vi "Actor Core.vi"(8 "error in":errorcluster, 11 "Monitor in":refnum<class "Classic Monitor.lvclass">) -> (0 "error out":errorcluster, 3 "Actor out":refnum<class "Actor.lvclass">)   [LabVIEW 2023, in "Monitored Actor.lvlib" / "Classic Monitor.lvclass"]
doc: "(<B>Filename</B>: Actor Framework.lvlib:Actor.lvclass:Actor Core.vi)\n\nReceives messages to the actor, reacts to them, and initiates any error handling that may shut the actor down.\n\nDescendant classes may override this VI to append parallel tasks for the actor to complete while it handles messages. Overrides use the Call Parent Method node."
uses:
  Classic Monitor.lvclass
  C:/Users/Public/Documents/Development/builds/Engine/Actor Framework.lvlibp/1abvi3w/vi.lib/ActorFramework/Actor/Actor.lvclass
  builds/Engine/Actor Framework.lvlibp/1abvi3w/vi.lib/ActorFramework/Actor/Actor.lvclass
  Monitor Data/Monitor Data.lvclass
  builds/Engine/Actor Framework.lvlibp/1abvi3w/vi.lib/ActorFramework/Message Enqueuer/Message Enqueuer.lvclass
  Classic Monitor.lvclass/Classic Monitor.ctl
  builds/Engine/Actor Framework.lvlibp/1abvi3w/vi.lib/ActorFramework/Time-Delayed Send Message/Time-Delay Override Options.ctl
  Orphan Detector/Orphan Detector/Orphan Detector.lvclass
  Actor Monitor/Actor Monitor Messages/Ping Actor Msg/Ping Actor Msg.lvclass
  C:/Users/Public/Documents/Development/builds/Engine/Actor Framework.lvlibp/1abvi3w/vi.lib/ActorFramework/Message/Message.lvclass
  Actor Monitor/Actor Monitor/Actor Monitor.lvclass
  Actor Monitor/Actor Monitor Messages/Manually Remove Actor Msg/Manually Remove Actor Msg.lvclass
  Monitor Messages/Log Messages Msg/Log Messages Msg.lvclass
  builds/Engine/Actor Framework.lvlibp/1abvi3w/vi.lib/ActorFramework/Stop Msg/Stop Msg.lvclass
  builds/Engine/Actor Framework.lvlibp
panel:
  in  "Monitored Actors":string[](tree)
  in  "Stop Actor":bool
  in  "Show Actor Core":bool
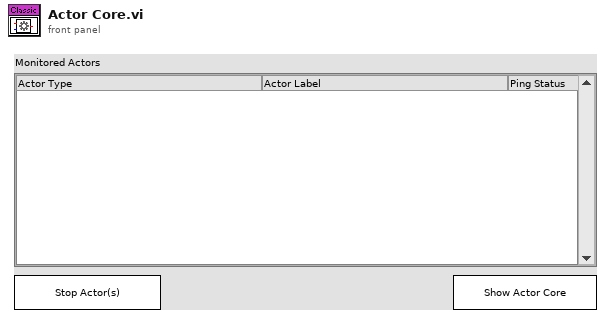
[diagram p1: front panel]
types:
  T1 = cluster{"Monitor Data":refnum<class "Monitor Data.lvclass">, "Changed Actor Q":refnum<class "Message Enqueuer.lvclass">}
  T2 = enum32{"Invalid", "Standard", "Closed", "Hidden", "Minimized", "Maximized"}
  T3 = cluster{"left":i16, "top":i16, "right":i16, "bottom":i16}
  T4 = typedef "Actor Framework.lvlibp/Time-Delay Override Options.ctl" = enum16{"Send next copy now", "Skip next scheduled copy", "Send next copy now and stop all further copies", "Stop all further copies"}
  T5 = enum8{"Enabled", "Disabled", "Disabled and Grayed Out"}
  T6 = typedef "LVRectTypeDef.ctl" = cluster{"Left":i16, "Top":i16, "Right":i16, "Bottom":i16}
  T7 = typedef "LVPoint32TypeDef.ctl" = cluster{"Horizontal":i32, "Vertical":i32}
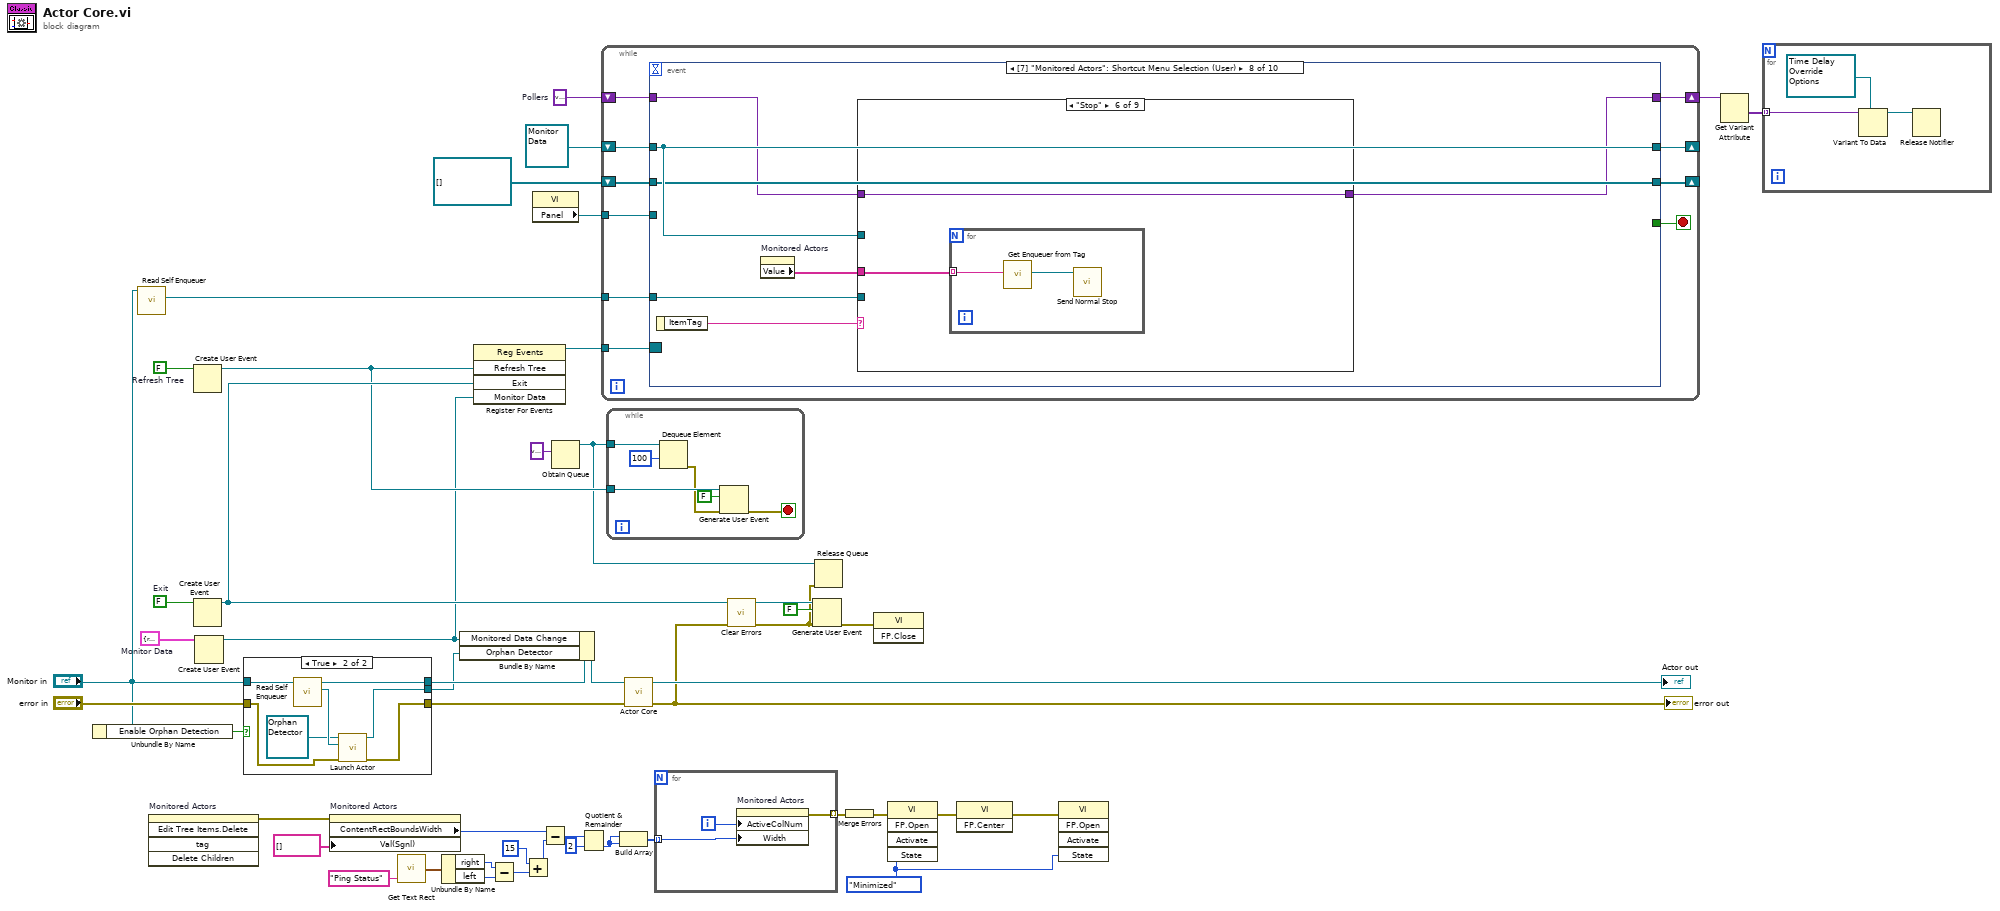
[diagram p0: block diagram]
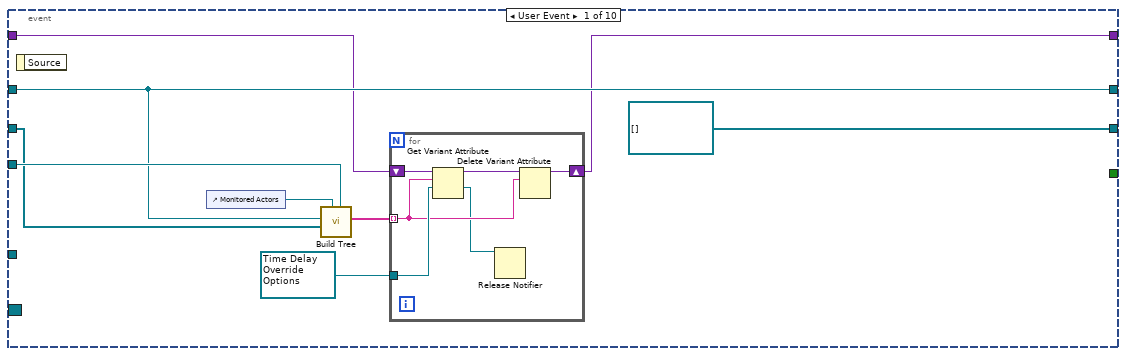
[diagram p3: hidden frame]
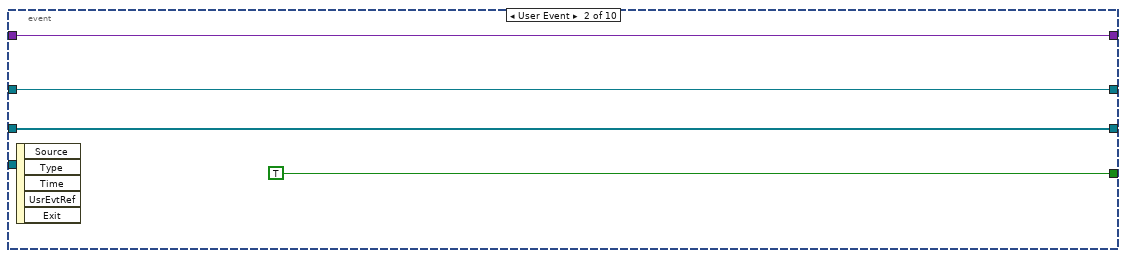
[diagram p4: hidden frame]
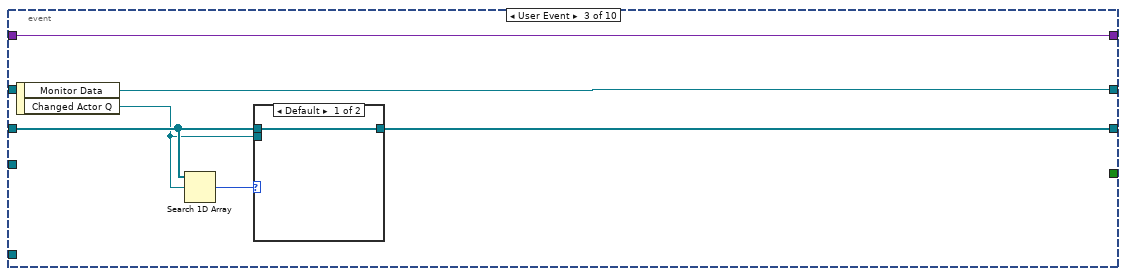
[diagram p5: hidden frame]
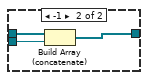
[diagram p6: hidden frame]
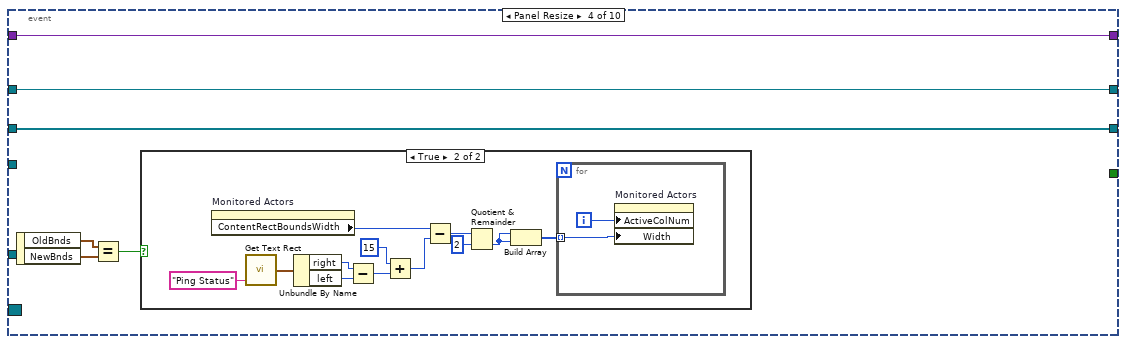
[diagram p7: hidden frame]
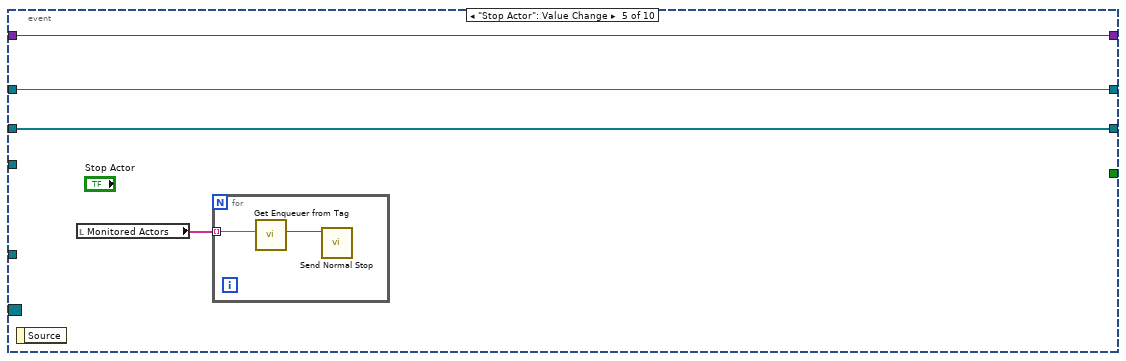
[diagram p9: hidden frame]
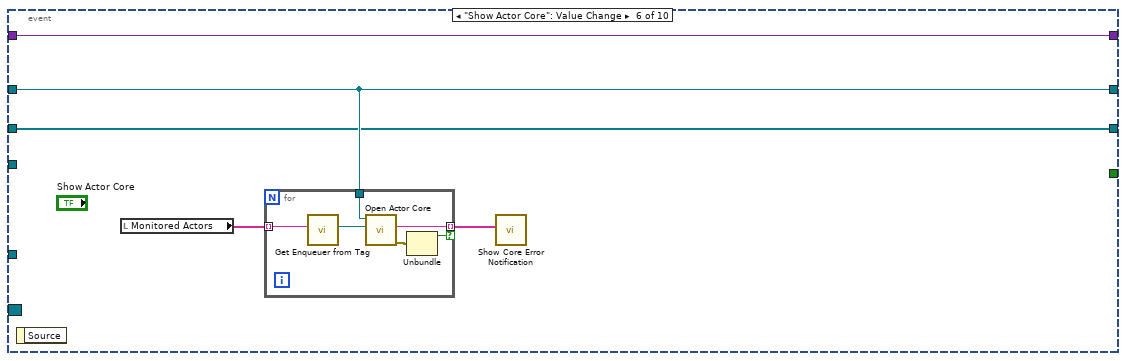
[diagram p10: hidden frame]
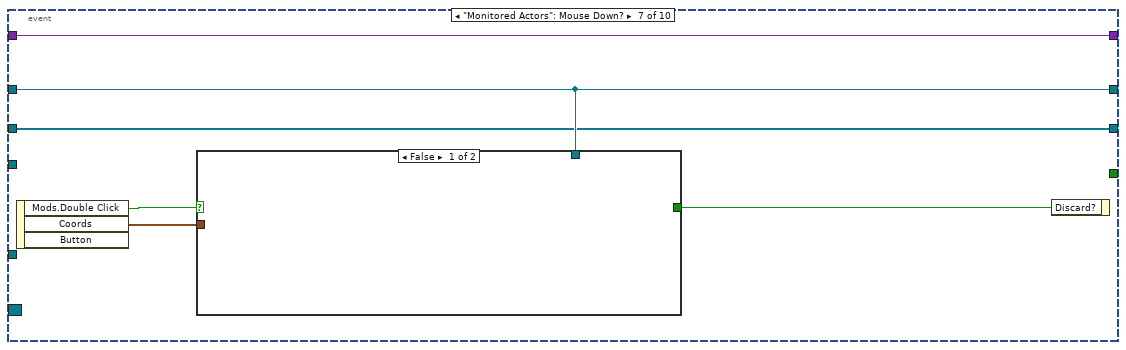
[diagram p11: hidden frame]
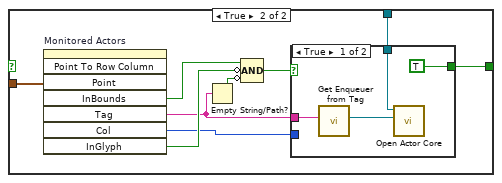
[diagram p12: hidden frame]
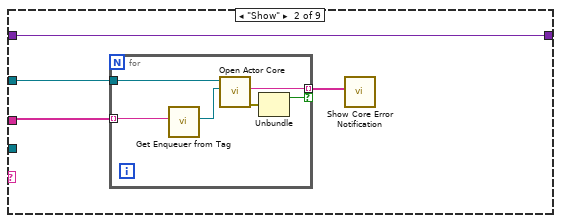
[diagram p15: hidden frame]
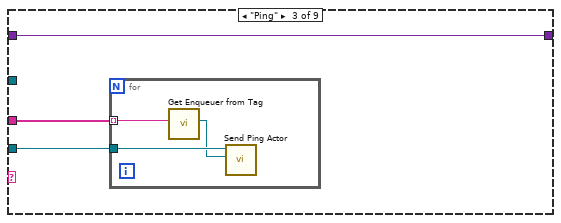
[diagram p16: hidden frame]
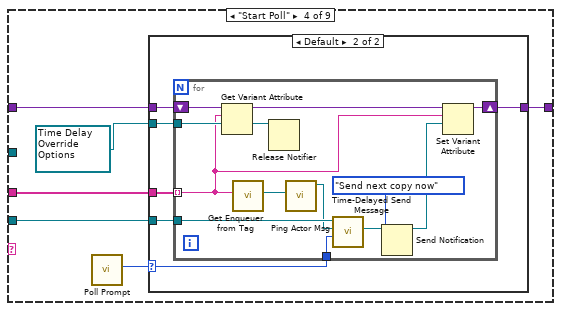
[diagram p17: hidden frame]
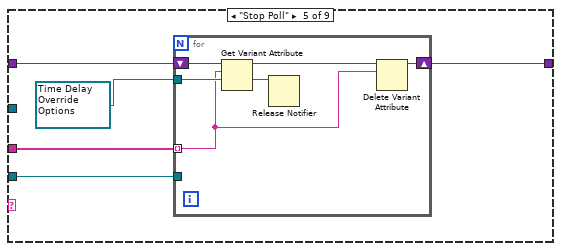
[diagram p19: hidden frame]
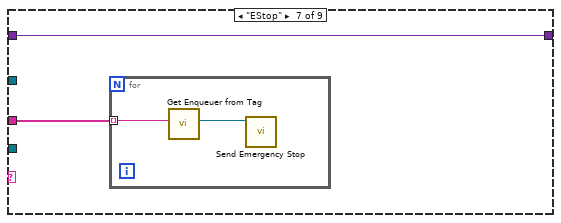
[diagram p20: hidden frame]
diagram:
  w4 = variant  # Pollers
  w15 = T1 {"Monitor Data"=refnum, "Changed Actor Q"=refnum}  # Monitor Data
  w20 = FALSE  # Refresh Tree
  w1 = T2."Minimized" ("State")
  w32 = FALSE  # Exit
  n1 = Unbundle By Name("Monitor in") -> ("Enable Orphan Detection"=w5:bool)
  n2 = call "Read Self Enqueuer.vi"("Actor"="Monitor in") -> ("Self Enqueuer"=w26:refnum<class "Message Enqueuer.lvclass">)  [unwired: 10 in]
  n3 = invoke on="Monitored Actors" class="Tree (strict)" method="Edit Tree Items.Delete"() -> (error out=w11:errorcluster)  [unwired: 5 in, 4 out]
  n4 = Create User Event(user event datatype=w20) -> (user event=w19:refnum<user-event>)  [unwired: 1 in, 1 out]
  n5 = Create User Event(user event datatype=w32) -> (user event=w31:refnum<user-event>)  [unwired: 1 in, 1 out]
  n6 = Create User Event(user event datatype=w15) -> (user event=w14:refnum<user-event>)  [unwired: 1 in, 1 out]
  n7 = case shown="True" w5 {
    tunnel: "error in" -> [w48 w51]
    tunnel: [w48 w50] -> w10
    tunnel: [w49 w54] -> w9
    tunnel: "Monitor in" -> [w49 w54]
    tunnel: [_ w52] -> w8
    frame False {
    }
    frame True {
      n8 = call "Read Self Enqueuer.vi"("Actor"=w54) -> ("Self Enqueuer"=w55:refnum<class "Message Enqueuer.lvclass">)  [unwired: 10 in]
      n9 = call "Launch Actor.vi"("error in (no error)"=w51, "Actor-to-Caller Enqueuer"=w55, "Actor"=refnum<class "Orphan Detector.lvclass"> refnum ("Classic Monitor.lvlib:Orphan Detector.lvclass")) -> ("error out"=w50:errorcluster, "Caller-To-Actor Enqueuer"=w52:refnum<class "Message Enqueuer.lvclass">)  [unwired: 7 in]
    }
  }
  n10 = property on="Monitored Actors" class="Tree (strict)"(error in=w11, "Val(Sgnl)"=string[] [] ("Value (Signaling)")) -> ("ContentRectBoundsWidth"=w45:i32)  [unwired: 1 in, 2 out]
  n11 = call <vilib>:"Get Text Rect.vi"("text"="Ping Status") -> ("rect"=w43:T3)  [unwired: 8 in]
  n12 = Unbundle By Name(w43) -> ("right"=w42:i16, "left"=w41:i16)
  n13 = Bundle By Name(cluster=w9, "Monitored Data Change"=w14, "Orphan Detector"=w8) -> (w29:refnum<class "Classic Monitor.lvclass">)
  n14 = register-events(w19, w31, w14) -> (reference out=w33:refnum<event-registration>)  [unwired: 2 in, 1 out]
  n15 = Subtract(x=w42, y=w41) -> (x-y=w40:i16)
  n16 = Add(x=i16 15, y=w40) -> (x+y=w37:i16)
  n17 = property class="VI"() -> ("Panel"=w27:refnum<vi>)  [unwired: 2 in, 2 out]
  n18 = Subtract(x=w45, y=w37) -> (x-y=w39:i32)
  n19 = Obtain Queue(element data type=variant) -> (queue out=w16:refnum<queue>)  [unwired: 4 in, 2 out]
  n20 = Quotient & Remainder(x=w39, y=2) -> (floor(x/y)=w35:i32)  [unwired: 1 out]
  n21 = while {
    tunnel: w33 -> [w65]
    shift-right: [w63] -> _
    shift-left: refnum<class "Monitor Data.lvclass"> refnum ("Monitor Data") -> [w62]
    tunnel: w27 -> [w61]
    tunnel: w26 -> [w60]
    shift-right: [w59] -> _
    shift-left: refnum<class "Message Enqueuer.lvclass">[] [] -> [w58]
    shift-right: [w57] -> w3
    shift-left: w4 -> [w56]
    stop <- w64 stop-if-true
    n22 = event shown="[7] \"Monitored Actors\": Shortcut Menu Selection (User)" {
      selector: w65 -> [_ _ _ _ _ _ _ _ _ _]
      dyn-events: _ -> [_ _ _ _ _ _ _ _ _ _]
      timeout: _ -> [_ _ _ _ _ _ _ _ _ _]
      tunnel: [_ TRUE _ _ _ _ _ _ _ _] -> w64
      tunnel: [w73 w83 w90 w100 w118 w124 w137 w157 w242 w259] -> w63
      tunnel: w62 -> [w73 w83 _ w100 w118 w124 w137 w157 w242 w259]
      tunnel: w61 -> [w74 _ _ _ _ _ _ _ _ _]
      tunnel: w60 -> [_ _ _ _ _ _ _ w154 _ _]
      tunnel: [refnum<class "Message Enqueuer.lvclass">[] [] w82 w89 w96 w116 w123 w133 w153 w243 w261] -> w59
      tunnel: w58 -> [w66 w82 w88 w96 w116 w123 w133 w153 w243 w261]
      tunnel: [w67 w81 w85 w95 w115 w121 w132 w151 w236 w252] -> w57
      tunnel: w56 -> [w68 w81 w85 w95 w115 w121 w132 w152 w236 w252]
      event User Event {
        w69 = refnum<notifier> refnum items=["Send next copy now", "Skip next scheduled copy", "Send next copy now and stop all further copies", "Stop all further copies"] ("Delivery Notifier")
        n23 = event-data() -> ()  [unwired: 1 in, 1 out]
        n24 = control-ref of="Monitored Actors"() -> (w72:refnum<vi>)
        n25 = call "Build Tree.vi"("Panel"=w74, "Tree"=w72, "Changed Actors"=w66, "Monitor Data"=w73) -> ("Stopped Actors"=w70:string[])  [unwired: 7 in]
        n26 = for {
          tunnel: w70 -> [w77] mode=indexing
          shift-right: [w76] -> w67
          shift-left: w68 -> [w80]
          tunnel: w69 -> [w79]
          n27 = Get Variant Attribute(Variant=w80, name=w77, default value (empty Variant)=w79) -> (duplicate Variant=w78:variant, value=w75:refnum<notifier>)  [unwired: 1 in, 2 out]
          n28 = Release Notifier(notifier=w75) -> ()  [unwired: 2 in, 3 out]
          n29 = Delete Variant Attribute(6:w77, 7:w78) -> (3:w76:variant)  [unwired: 1 in, 2 out]
        }
      }
      event User Event {
        n30 = event-data() -> ()  [unwired: 1 in, 5 out]
      }
      event User Event {
        n31 = event-data() -> ("Monitor Data"=w90:refnum<class "Monitor Data.lvclass">, "Changed Actor Q"=w87:refnum<class "Message Enqueuer.lvclass">)  [unwired: 1 in]
        n32 = Search 1D Array(1D array=w88, element=w87) -> (index of element=w86:i32)  [unwired: 1 in]
        n33 = case shown="Default" w86 {
          tunnel: [w91 w94] -> w89
          tunnel: w88 -> [w91 w93]
          tunnel: w87 -> [_ w92]
          frame Default {
          }
          frame -1 {
            n34 = Build Array (concatenate)(w93, w92) -> (w94:refnum<class "Message Enqueuer.lvclass">[])
          }
        }
      }
      event Panel Resize {
        n35 = event-data() -> ("OldBnds"=w99:T6, "NewBnds"=w98:T6)  [unwired: 1 in]
        n36 = Equal?(x=w99, y=w98) -> (x = y?=w97:bool)
        n37 = case shown="True" w97 {
          frame False {
          }
          frame True {
            n38 = property on="Monitored Actors" class="Tree (strict)"() -> ("ContentRectBoundsWidth"=w101:i32)  [unwired: 2 in, 2 out]
            n39 = call <vilib>:"Get Text Rect.vi"("text"="Ping Status") -> ("rect"=w103:T3)  [unwired: 8 in]
            n40 = Unbundle By Name(w103) -> ("right"=w104:i16, "left"=w105:i16)
            n41 = Subtract(x=w104, y=w105) -> (x-y=w106:i16)
            n42 = Add(x=i16 15, y=w106) -> (x+y=w109:i16)
            n43 = Subtract(x=w101, y=w109) -> (x-y=w107:i32)
            n44 = Quotient & Remainder(x=w107, y=2) -> (floor(x/y)=w111:i32)  [unwired: 1 out]
            n45 = Build Array(w111, w111) -> (w112:i32[])
            n46 = for {
              tunnel: w112 -> [w113] mode=indexing
              i -> [w114]
              n47 = property on="Monitored Actors" class="Tree (strict)"("ActiveColNum"=w114, "Width"=w113) -> ()  [unwired: 2 in, 2 out]
            }
          }
        }
      }
      event "Stop Actor": Value Change {
        n48 = event-data() -> ()  [unwired: 1 in, 1 out]
        n49 = local read "Monitored Actors"() -> (w117:string[])
        n50 = for {
          tunnel: w117 -> [w120] mode=indexing
          n51 = call "Get Enqueuer from Tag.vi"("Tag"=w120) -> ("Enqueuer"=w119:refnum<class "Message Enqueuer.lvclass">)  [unwired: 10 in]
          n52 = call "Send Normal Stop.vi"("Message Enqueuer"=w119) -> ()  [unwired: 10 in, 1 out]
        }
      }
      event "Show Actor Core": Value Change {
        n53 = event-data() -> ()  [unwired: 1 in, 1 out]
        n54 = local read "Monitored Actors"() -> (w125:string[])
        n55 = for {
          tunnel: w125 -> [w131] mode=indexing
          tunnel: w124 -> [w130]
          tunnel: [w128] -> w122 mode=indexing if=w126
          n56 = call "Get Enqueuer from Tag.vi"("Tag"=w131) -> ("Enqueuer"=w129:refnum<class "Message Enqueuer.lvclass">)  [unwired: 10 in]
          n57 = call "Open Actor Core.vi"("Actor's Self Q"=w129, "Monitor Data"=w130) -> ("error out"=w127:errorcluster, "Actor Core VI"=w128:string)  [unwired: 8 in]
          n58 = Unbundle(w127) -> ("status"=w126:bool)  [unwired: 2 out]
        }
        n59 = call "Show Core Error Notification.vi"("Error VIs"=w122) -> ()  [unwired: 11 in]
      }
      event "Monitored Actors": Mouse Down? {
        n60 = event-data() -> ("Mods.Double Click"=w136:bool, "Coords"=w135:T7)  [unwired: 1 in, 1 out]
        n61 = case shown="False" w136 {
          tunnel: w137 -> [_ w146]
          tunnel: w135 -> [_ w145]
          tunnel: [_ w142] -> w134
          frame False {
          }
          frame True {
            n62 = invoke on="Monitored Actors" class="Tree (strict)" method="Point To Row Column"("Point"=w145) -> ("InBounds"=w144:bool, "Tag"=w139:string, "Col"=w138:i32, "InGlyph"=w143:bool)  [unwired: 7 in, 4 out]
            n63 = Empty String/Path?(string/path=w139) -> (empty?=w140:bool)
            n64 = Compound Arithmetic op=AND(w144, invert w143, invert w140) -> (w141:bool)
            n65 = case shown="True" w141 {
              tunnel: w146 -> [w148 _]
              tunnel: [TRUE _] -> w142
              tunnel: w139 -> [w150 _]
              tunnel: w138 -> [_ _]
              frame True {
                n66 = call "Get Enqueuer from Tag.vi"("Tag"=w150) -> ("Enqueuer"=w147:refnum<class "Message Enqueuer.lvclass">)  [unwired: 10 in]
                n67 = call "Open Actor Core.vi"("Actor's Self Q"=w147, "Monitor Data"=w148) -> ()  [unwired: 8 in, 2 out]
              }
              frame False {
              }
            }
          }
        }
        n68 = event-data("Discard?"=w134) -> ()  [unwired: 1 in, 1 out]
      }
      event "Monitored Actors": Shortcut Menu Selection (User) {
        n69 = event-data() -> ("ItemTag"=w156:string)  [unwired: 1 in]
        n70 = property on="Monitored Actors" class="Tree (strict)"() -> ("Value"=w155:string[])  [unwired: 2 in, 2 out]
        n71 = case shown="\"Stop\"" w156 {
          tunnel: w157 -> [_ w161 _ _ _ _ _ _ _]
          tunnel: w155 -> [_ w162 w171 w180 w205 w213 w217 w224 w232]
          tunnel: w154 -> [_ _ w170 w179 w204 _ _ w223 w231]
          tunnel: w152 -> [w158 w159 w169 w178 w203 w212 w216 w220 w230]
          tunnel: [w158 w159 w169 w177 w202 w212 w216 w220 w230] -> w151
          frame Default {
          }
          frame "Show" {
            n72 = for {
              tunnel: w162 -> [w168] mode=indexing
              tunnel: w161 -> [w167]
              tunnel: [w165] -> w160 mode=indexing if=w163
              n73 = call "Get Enqueuer from Tag.vi"("Tag"=w168) -> ("Enqueuer"=w166:refnum<class "Message Enqueuer.lvclass">)  [unwired: 10 in]
              n74 = call "Open Actor Core.vi"("Actor's Self Q"=w166, "Monitor Data"=w167) -> ("error out"=w164:errorcluster, "Actor Core VI"=w165:string)  [unwired: 8 in]
              n75 = Unbundle(w164) -> ("status"=w163:bool)  [unwired: 2 out]
            }
            n76 = call "Show Core Error Notification.vi"("Error VIs"=w160) -> ()  [unwired: 11 in]
          }
          frame "Ping" {
            n77 = for {
              tunnel: w171 -> [w174] mode=indexing
              tunnel: w170 -> [w173]
              n78 = call "Get Enqueuer from Tag.vi"("Tag"=w174) -> ("Enqueuer"=w172:refnum<class "Message Enqueuer.lvclass">)  [unwired: 10 in]
              n79 = call "Send Ping Actor.vi"("Actor"=w172, "Message Enqueuer in"=w173) -> ()  [unwired: 8 in, 2 out]
            }
          }
          frame "Start Poll" {
            w176 = refnum<notifier> refnum items=["Send next copy now", "Skip next scheduled copy", "Send next copy now and stop all further copies", "Stop all further copies"] ("Delivery Notifier")
            n80 = call "Poll Prompt.vi"() -> ("Period"=w175:i32)  [unwired: 10 in, 1 out]
            n81 = case shown="Default" w175 {
              selector: w175 -> [_ w182]
              tunnel: w180 -> [_ w187]
              tunnel: w179 -> [_ w186]
              tunnel: w178 -> [w181 w185]
              tunnel: [w181 w184] -> w177
              tunnel: w176 -> [_ w183]
              frame -1 {
              }
              frame Default {
                n82 = for {
                  tunnel: w187 -> [w191] mode=indexing
                  tunnel: w186 -> [w200]
                  shift-right: [w193] -> w184
                  shift-left: w185 -> [w197]
                  tunnel: w183 -> [w195]
                  tunnel: w182 -> [w190]
                  n83 = Get Variant Attribute(Variant=w197, name=w191, default value (empty Variant)=w195) -> (duplicate Variant=w196:variant, value=w194:refnum<notifier>)  [unwired: 1 in, 2 out]
                  n84 = call "Get Enqueuer from Tag.vi"("Tag"=w191) -> ("Enqueuer"=w199:refnum<class "Message Enqueuer.lvclass">)  [unwired: 10 in]
                  n85 = Release Notifier(notifier=w194) -> ()  [unwired: 2 in, 3 out]
                  n86 = call "Ping Actor Msg.vi"("Actor"=w199) -> ("Ping Actor Msg out"=w198:refnum<class "Ping Actor Msg.lvclass">)  [unwired: 9 in, 1 out]
                  n87 = call "Time-Delayed Send Message.vi"("Milliseconds To Wait"=w190, "Message"=w198, "Message Enqueuer"=w200) -> ("Delivery Notifier"=w192:refnum<notifier>)  [unwired: 7 in, 1 out]
                  n88 = Send Notification(notification=Time-Delay_Override_Options."Send next copy now" ("Time Delay Override Options"), notifier=w192) -> (notifier out=w189:refnum<notifier>)  [unwired: 1 in, 1 out]
                  n89 = Set Variant Attribute(Variant=w196, name=w191, value=w189) -> (Variant out=w193:variant)  [unwired: 1 in, 2 out]
                }
              }
            }
          }
          frame "Stop Poll" {
            w201 = refnum<notifier> refnum items=["Send next copy now", "Skip next scheduled copy", "Send next copy now and stop all further copies", "Stop all further copies"] ("Delivery Notifier")
            n90 = for {
              tunnel: w205 -> [w206] mode=indexing
              tunnel: w204 -> [_]
              shift-right: [w207] -> w202
              shift-left: w203 -> [w211]
              tunnel: w201 -> [w209]
              n91 = Get Variant Attribute(Variant=w211, name=w206, default value (empty Variant)=w209) -> (duplicate Variant=w210:variant, value=w208:refnum<notifier>)  [unwired: 1 in, 2 out]
              n92 = Release Notifier(notifier=w208) -> ()  [unwired: 2 in, 3 out]
              n93 = Delete Variant Attribute(6:w206, 7:w210) -> (3:w207:variant)  [unwired: 1 in, 2 out]
            }
          }
          frame "Stop" {
            n94 = for {
              tunnel: w213 -> [w215] mode=indexing
              n95 = call "Get Enqueuer from Tag.vi"("Tag"=w215) -> ("Enqueuer"=w214:refnum<class "Message Enqueuer.lvclass">)  [unwired: 10 in]
              n96 = call "Send Normal Stop.vi"("Message Enqueuer"=w214) -> ()  [unwired: 10 in, 1 out]
            }
          }
          frame "EStop" {
            n97 = for {
              tunnel: w217 -> [w219] mode=indexing
              n98 = call "Get Enqueuer from Tag.vi"("Tag"=w219) -> ("Enqueuer"=w218:refnum<class "Message Enqueuer.lvclass">)  [unwired: 10 in]
              n99 = call "Send Emergency Stop.vi"("Message Enqueuer"=w218) -> ()  [unwired: 10 in, 1 out]
            }
          }
          frame "Remove" {
            n100 = Two Button Dialog(message="Warning: Manually removing actors from list can lead to inconsitancies between the monitor and the actual state.\n\n Only do this if you're sure the actor has been aborted manually.") -> (T button?=w221:bool)  [unwired: 2 in]
            n101 = case shown="True" w221 {
              tunnel: w224 -> [_ w226]
              tunnel: w223 -> [_ w225]
              frame False {
              }
              frame True {
                n102 = for {
                  tunnel: w226 -> [w229] mode=indexing
                  tunnel: w225 -> [w227]
                  n103 = call "Get Enqueuer from Tag.vi"("Tag"=w229) -> ("Enqueuer"=w228:refnum<class "Message Enqueuer.lvclass">)  [unwired: 10 in]
                  n104 = call "Send Manually Remove Actor.vi"("Actor's Q"=w228, "Message Enqueuer in"=w227) -> ()  [unwired: 8 in, 2 out]
                }
              }
            }
          }
          frame "Logging" {
            n105 = for {
              tunnel: w232 -> [w235] mode=indexing
              tunnel: w231 -> [w234]
              n106 = call "Get Enqueuer from Tag.vi"("Tag"=w235) -> ("Enqueuer"=w233:refnum<class "Message Enqueuer.lvclass">)  [unwired: 10 in]
              n107 = call "Send Log Messages.vi"("Actor to Log"=w233, "Message Enqueuer in"=w234) -> ()  [unwired: 8 in, 2 out]
            }
          }
        }
      }
      event "Monitored Actors": Value Change {
        n108 = event-data() -> ()  [unwired: 1 in, 1 out]
        n109 = Empty Array?(array="Monitored Actors") -> (empty?=w240:bool)
        n110 = Select(t=T5."Disabled and Grayed Out" ("Disabled"), s=w240, f=T5."Enabled") -> (s? t:f=w237:T5)
        n111 = property on="Stop Actor" class="Bool"("DisabledEnum"=w237) -> ()  [unwired: 2 in, 2 out]
        n112 = property on="Show Actor Core" class="Bool"("DisabledEnum"=w237) -> ()  [unwired: 2 in, 2 out]
      }
      event "Monitored Actors": Shortcut Menu Activation? {
        n113 = event-data() -> ("MenuRef"=w260:refnum<k9>, "Coords"=w258:T7)  [unwired: 1 in]
        n114 = disable-structure shown="Disable_Msg_Log==True" {
          disable-tunnel: w260 -> [w271 w272]
          disable-tunnel: [w268 w272] -> w250
          frame condition #0 {
            n115 = Set Menu Item Info(7:"Logging" ("item name"), 9:FALSE ("enabled"), 11:w271) -> (3:w268:refnum<k9>)  [unwired: 4 in, 1 out]
          }
          frame condition #1 (active) {
          }
        }
        n116 = invoke on="Monitored Actors" class="Tree (strict)" method="Point To Row Column"("Point"=w258) -> ("Tag"=w257:string)  [unwired: 7 in, 7 out]
        n117 = property on="Monitored Actors" class="Tree (strict)"() -> ("Value"=w254:string[])  [unwired: 2 in, 2 out]
        n118 = Search 1D Array(1D array=w254, element=w257) -> (index of element=w255:i32)  [unwired: 1 in]
        n119 = Build Array(w257) -> (w256:string[])
        n120 = case shown="-1" w255 {
          tunnel: w256 -> [_ w267]
          tunnel: w254 -> [w265 w266]
          tunnel: [w265 w266] -> w253
          frame Default {
          }
          frame -1 {
            n121 = property on="Monitored Actors" class="Tree (strict)"("Val(Sgnl)"=w267) -> ()  [unwired: 2 in, 2 out]
          }
        }
        n122 = for {
          tunnel: w253 -> [w263] mode=indexing
          tunnel: w252 -> [w264]
          tunnel: [w262] -> w247 mode=indexing
          n123 = Get Variant Attribute(Variant=w264, name=w263) -> (found=w262:bool)  [unwired: 2 in, 3 out]
        }
        n124 = Or Array Elements(Boolean array=w247) -> (logical OR=w244:bool)
        n125 = And Array Elements(Boolean array=w247) -> (logical AND=w246:bool)
        n126 = Not(x=w246) -> (.not. x?=w245:bool)
        n127 = Set Menu Item Info(7:"Stop Poll" ("item name"), 9:w244, 11:w250) -> (3:w249:refnum<k9>)  [unwired: 4 in, 1 out]
        n128 = Set Menu Item Info(7:"Start Poll" ("item tag"), 9:w245, 11:w249) -> ()  [unwired: 4 in, 2 out]
        n129 = event-data() -> ()  [unwired: 2 in, 1 out]
      }
    }
  }
  n130 = while {
    tunnel: w16 -> [w277]
    tunnel: w19 -> [w276]
    stop <- w274 stop-if-true
    n131 = Dequeue Element(queue=w277, timeout in ms (-1)=100) -> (error out=w275:errorcluster)  [unwired: 1 in, 3 out]
    n132 = Generate User Event(user event=w276, event data cluster=FALSE ("event data"), error in=w275) -> (error out=w274:errorcluster)  [unwired: 1 in, 1 out]
  }
  n133 = Build Array(w35, w35) -> (w34:i32[])
  n134 = call-parent "Actor Core.vi"("error in"=w10, "Actor in"=w29) -> ("error out"=w30:errorcluster, "Actor out"=→"Actor out":refnum<class "Actor.lvclass">)  [unwired: 8 in]
  "error out" <- w30
  n135 = for {
    tunnel: w34 -> [w280] mode=indexing
    tunnel: [w279] -> w25 mode=indexing
    i -> [w281]
    n136 = property on="Monitored Actors" class="Tree (strict)"("ActiveColNum"=w281, "Width"=w280) -> (error out=w279:errorcluster)  [unwired: 2 in, 1 out]
  }
  n137 = call <vilib>:"Clear Errors.vi"("error in (no error)"=w30) -> ("error out"=w17:errorcluster)  [unwired: 5 in, 1 out]
  n138 = Generate User Event(user event=w31, event data cluster=FALSE ("event data"), error in=w17) -> (error out=w24:errorcluster)  [unwired: 1 in, 1 out]
  n139 = Release Queue(queue=w16, error in (no error)=w17) -> ()  [unwired: 1 in, 3 out]
  n140 = Merge Errors(w25) -> (w22:errorcluster)
  n141 = invoke class="VI" method="FP.Close"(error in=w24) -> ()  [unwired: 2 in, 3 out]
  n142 = invoke class="VI" method="FP.Open"(error in=w22, "State"=w1) -> (error out=w23:errorcluster)  [unwired: 3 in, 4 out]
  n143 = invoke class="VI" method="FP.Center"(error in=w23) -> (error out=w21:errorcluster)  [unwired: 2 in, 2 out]
  n144 = invoke class="VI" method="FP.Open"(error in=w21, "State"=w1) -> ()  [unwired: 3 in, 5 out]
  n145 = Get Variant Attribute(Variant=w3) -> (values=w2:variant[])  [unwired: 3 in, 3 out]
  n146 = for {
    tunnel: w2 -> [w284] mode=indexing
    w283 = refnum<notifier> refnum items=["Send next copy now", "Skip next scheduled copy", "Send next copy now and stop all further copies", "Stop all further copies"] ("Delivery Notifier")
    n147 = Variant To Data(type=w283, Variant=w284) -> (data=w282:refnum<notifier>)  [unwired: 1 in, 1 out]
    n148 = Release Notifier(notifier=w282) -> ()  [unwired: 2 in, 3 out]
  }
